vi "Set into drive mode.vi"(8 "error in (no error)":errorcluster, 11 "SDO object in":refnum<k20>) -> (0 "error out":errorcluster, 3 "SDO object out":refnum<k20>)   [LabVIEW 2016]
uses:
  Set Controlword.vi
panel:
  out "completion codes":u32[](array[numeric])
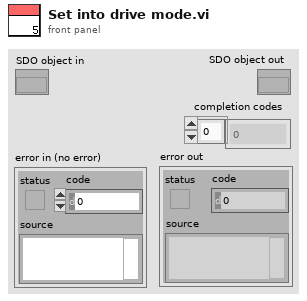
[diagram p1: front panel]
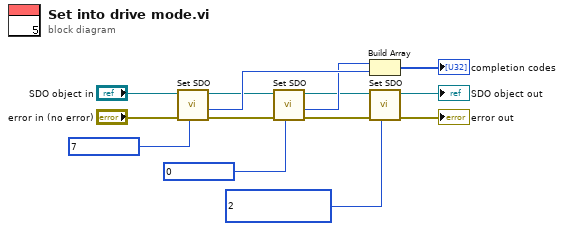
[diagram p0: block diagram]
diagram:
  n1 = call-poly "Set SDO.vi"("Controlword"=u8 7, "error in (no error)"="error in (no error)", "SDO object in"="SDO object in") -> ("error out"=w8:errorcluster, "completion code"=w14:u32, "SDO object out"=w10:refnum<k20>)  [unwired: 6 in]
  n2 = call-poly "Set SDO.vi"("Controlword"=u8 0, "error in (no error)"=w8, "SDO object in"=w10) -> ("error out"=w4:errorcluster, "completion code"=w13:u32, "SDO object out"=w6:refnum<k20>)  [unwired: 6 in]
  n3 = Build Array(w13, w14) -> (→"completion codes":u32[])
  n4 = call-poly "Set SDO.vi"("Controlword"=u8 2, "error in (no error)"=w4, "SDO object in"=w6) -> ("error out"=→"error out":errorcluster, "SDO object out"=→"SDO object out":refnum<k20>)  [unwired: 6 in, 1 out]
